vi "Display Warnings.vi"(8 "error in (no error)":errorcluster, 10 "build":bool, 11 "AB_UI_Frmwk_Installer in":refnum<class "AB_UI_Frmwk_Installer.lvclass">) -> (0 "error out":errorcluster, 2 "continue?":bool, 3 "AB_UI_Frmwk_Installer out":refnum<class "AB_UI_Frmwk_Installer.lvclass">)   [LabVIEW 2020, in "AB_UI_Frmwk_Installer.lvclass"]
uses:
  <vilib>/AppBuilder/IB_Classes/Installer/UI/AB_UI_Frmwk_Installer.lvclass
  <vilib>/AppBuilder/IB_Classes/Installer/UI/AB_UI_Frmwk_Installer.lvclass/AB_UI_Frmwk_Installer.ctl
  <resource>/Framework/Providers/Builds/AppBuilder/AB_UI_Frmwk.lvclass
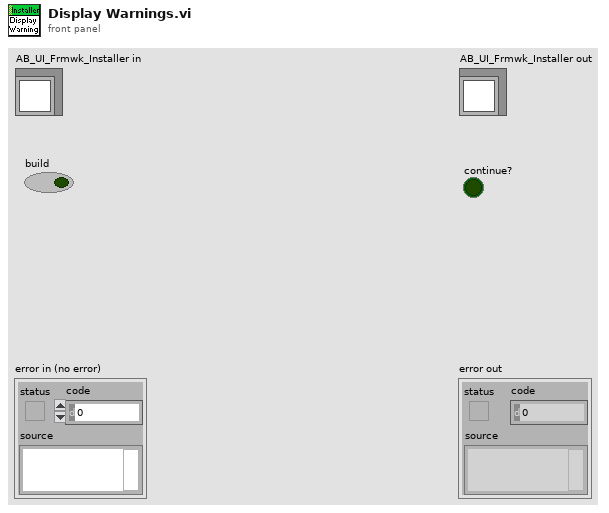
[diagram p1: front panel]
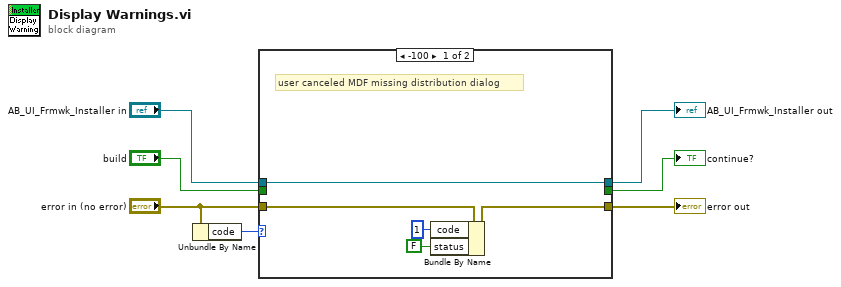
[diagram p0: block diagram]
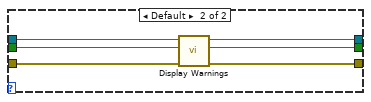
[diagram p2: hidden frame]
diagram:
  n1 = Unbundle By Name("error in (no error)") -> ("code"=w1:i32)
  n2 = case shown="-100" w1 {
    tunnel: [w10 w18] -> w7
    tunnel: [_ w17] -> w6
    tunnel: [w12 w16] -> w5
    tunnel: "build" -> [_ w15]
    tunnel: "AB_UI_Frmwk_Installer in" -> [w12 w14]
    tunnel: "error in (no error)" -> [w11 w13]
    frame -100 {
      # "user canceled MDF missing distribution dialog"
      n3 = Bundle By Name(cluster=w11, "code"=1, "status"=FALSE) -> (w10:errorcluster)
    }
    frame Default {
      n4 = call-parent "Display Warnings.vi"("error in (no error)"=w13, "build"=w15, "AB_UI_Frmwk in"=w14) -> ("error out"=w18:errorcluster, "continue?"=w17:bool, "AB_UI_Frmwk out"=w16:refnum<class "AB_UI_Frmwk_Installer.lvclass">)  [unwired: 6 in]
    }
  }
  "error out" <- w7
  "AB_UI_Frmwk_Installer out" <- w5
  "continue?" <- w6
